vi "Insert Status Data.vi"(0 "OutputData in":dbl[](array[numeric]), 5 "Late?":bool, 7 "error in (no error)":errorcluster, 9 "Read Duration":u32, 11 "Write Duration":u32, 12 "Status Channel Indexes":i32[](array[numeric])) -> (4 "OutputData out":dbl[](array[numeric]))   [LabVIEW 2010, in "RefMem PtByPt Custom Device.lvlib"]
uses:
  RefMem PtByPt Custom Device.lvlib
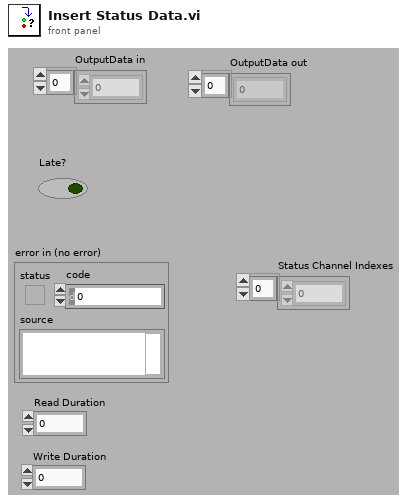
[diagram p1: front panel]
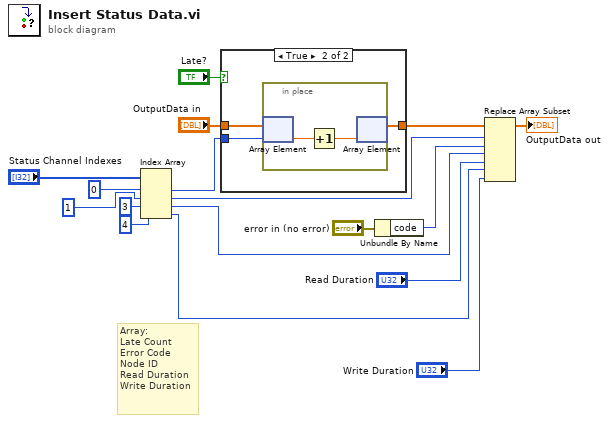
[diagram p0: block diagram]
diagram:
  # "Array:\nLate Count\nError Code\nNode ID\nRead Duration\nWrite Duration"
  n1 = Index Array(array="Status Channel Indexes", index #1=0 ("index"), index #2=1 ("index"), index #3=3 ("index"), index #4=4 ("index")) -> (element #1=w9:i32, element #2=w8:i32, element #3=w7:i32, element #4=w6:i32)
  n2 = case shown="True" "Late?" {
    tunnel: "OutputData in" -> [w18 w21]
    tunnel: [w18 w20] -> w14
    tunnel: w9 -> [_ w19]
    frame False {
    }
    frame True {
      n3 = in-place {
        n4 = in-place-array #1(w21, w19) -> (w23:dbl)
        n5 = Increment(x=w23) -> (x+1=w22:dbl)
        n6 = in-place-array #1(w22) -> (w20:dbl[])  [unwired: 1 out]
      }
    }
  }
  n7 = Unbundle By Name("error in (no error)") -> ("code"=w12:i32)
  n8 = Replace Array Subset(array=w14, new element #1=w12, index #1=w8, new element #2="Read Duration", index #2=w7, new element #3="Write Duration", index #3=w6) -> (→"OutputData out":dbl[])
